vi "potentiometer.vi"() -> ()   [LabVIEW 2017]
panel:
  in  "Tab Control":enum32{"Page 1", "Page 2"}(tab)
  out "Waveform Chart":dynamicdata(graph)
  in  "stop":bool
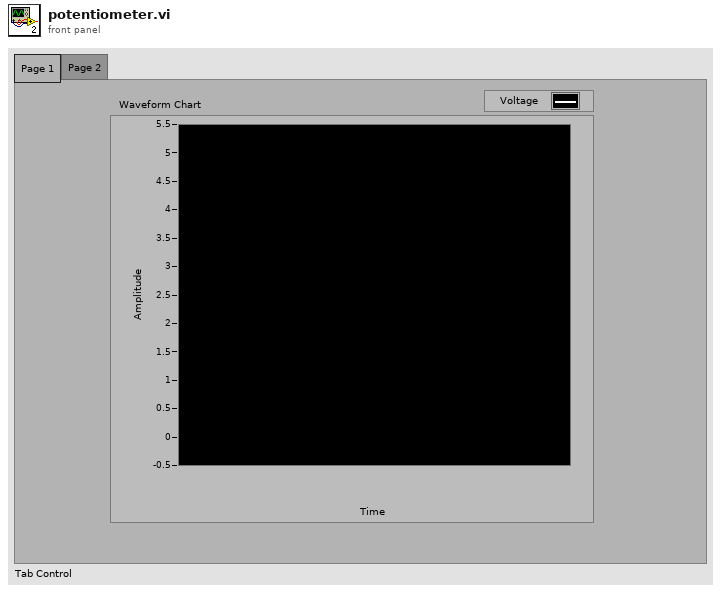
[diagram p1: front panel]
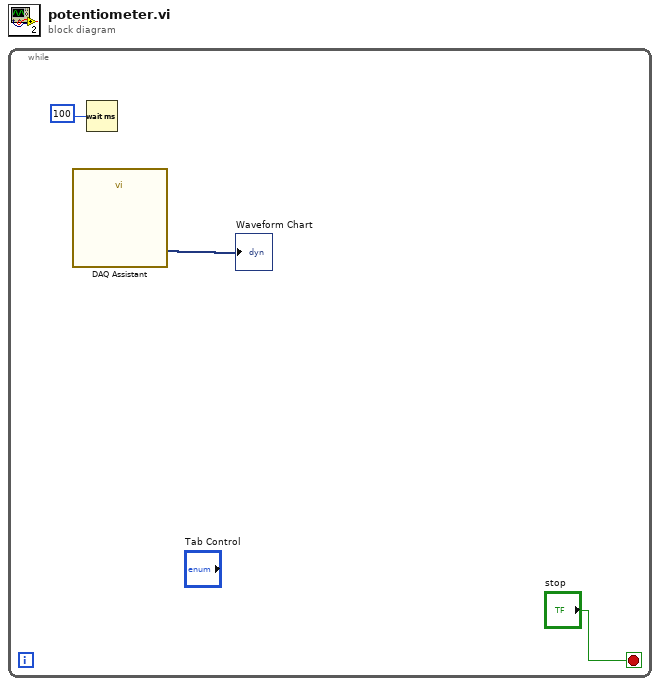
[diagram p0: block diagram]
diagram:
  n1 = while {
    stop <- "stop" stop-if-true
    n2 = call "DAQ Assistant"() -> ("data"=→"Waveform Chart":dynamicdata)  [unwired: 17 in, 2 out]
    n3 = Wait (ms)(milliseconds to wait=100) -> ()  [unwired: 1 out]
  }
